vi "MOPX1 Crossover.vi"(6 "Job Selection Rule":T1, 7 "Parent 1 Schedule":u16[](array[numeric]), 8 "error in (no error)":errorcluster, 9 "Parent 2 Schedule":u16[](array[numeric]), 10 "OSSP_Problem In":refnum<class "OSSP_Problem.lvclass">, 11 "GA in":refnum<class "GA.lvclass">) -> (0 "error out":errorcluster, 1 "Child 1":T2, 2 "OSSP_Problem out":refnum<class "OSSP_Problem.lvclass">, 3 "GA out":refnum<class "GA.lvclass">, 4 "Child 2":T2)   [LabVIEW 2013, in "GA.lvclass"]
uses:
  GA.lvclass
  OSSP_Problem.lvclass
  Controls/Solution_GA.ctl
  Controls/MPOX1 Operation Selection Rule.ctl
  GA.lvclass/GA.ctl
  OSSP_Problem.lvclass/OSSP_Problem.ctl
  GanntChart_Class/Operation to Machine Job Tuple.vi
  GanntChart_Class/Check Other Machines for Schedule Time.vi
  GanntChart_Class/Schedule Job.vi
  GanntChart_Class/Find Gaps on Particular Machine.vi
  GanntChart_Class/Increment Number of Jobs on Machine.vi
  GanntChart_Class/Find Job On Other Machines.vi
  GanntChart.lvclass
panel:
  out "Child 2 Schedule":u16[](array[numeric])
  out "Child 1 Schedule":u16[](array[numeric])
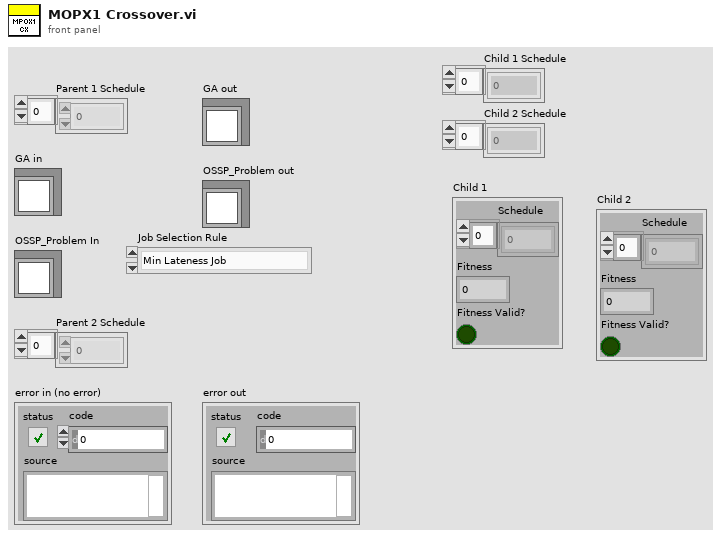
[diagram p1: front panel]
types:
  T1 = typedef "GA.lvclass/MPOX1 Operation Selection Rule.ctl" = enum16{"Min Lateness Job", "Random Job"}
  T2 = typedef "Solution_GA.ctl" = cluster{"Schedule":u16[], "Fitness":u16, "Fitness Valid?":bool}
  T3 = typedef "Scheduler Type.ctl" = enum16{"Non Delay Scheduler", "GT Active Scheduler", "FIFO Scheduler"}
  T4 = typedef "Objective.ctl" = enum16{"Makespan", "Total Tardiness"}
  T5 = typedef "GanntChart_Element.ctl" = cluster{"Operation Number":i32, "Job Number":i32, "Start Time":i32, "Procesing Time":u16, "End Time":i32}
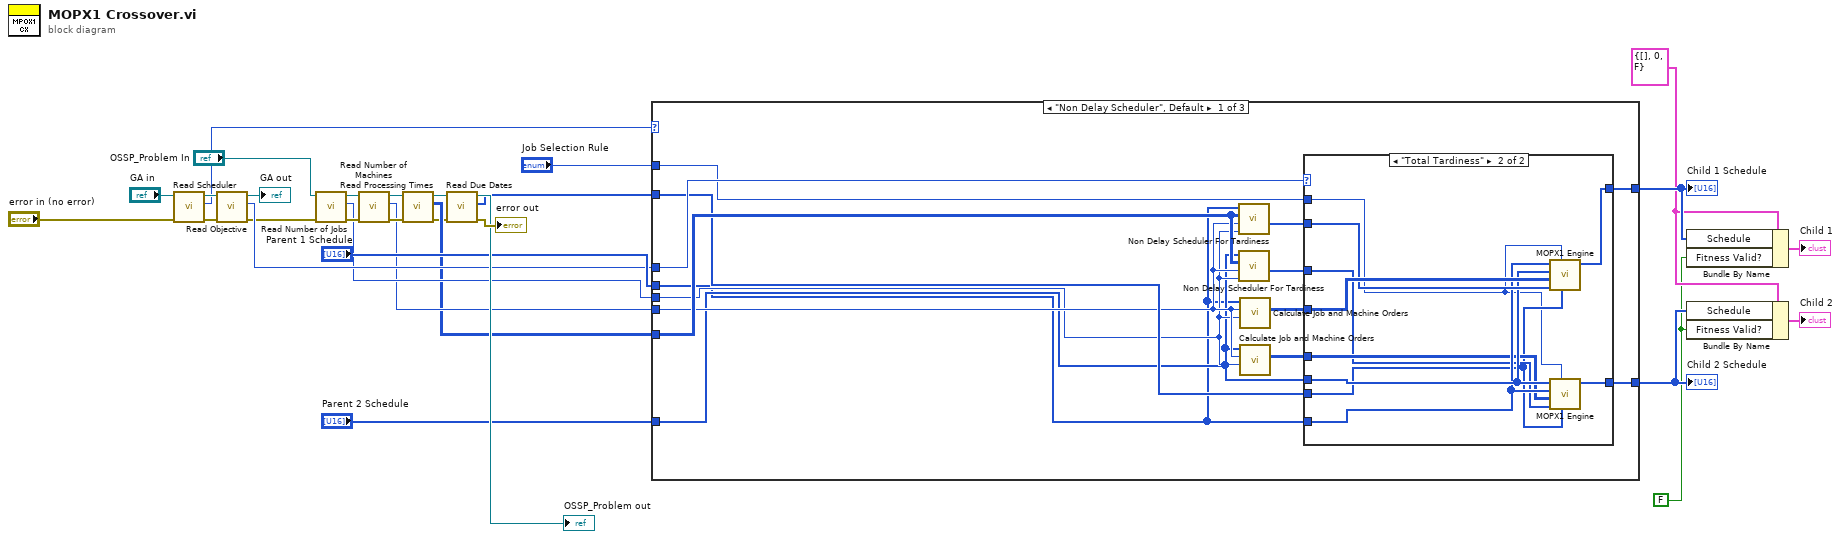
[diagram p0: block diagram]
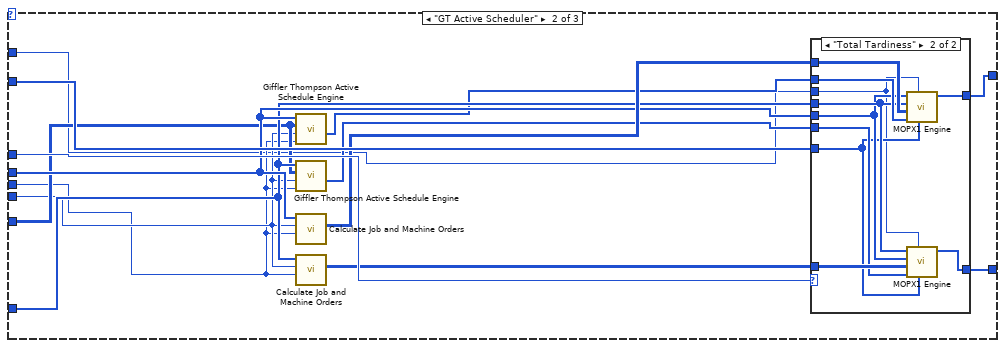
[diagram p3: hidden frame]
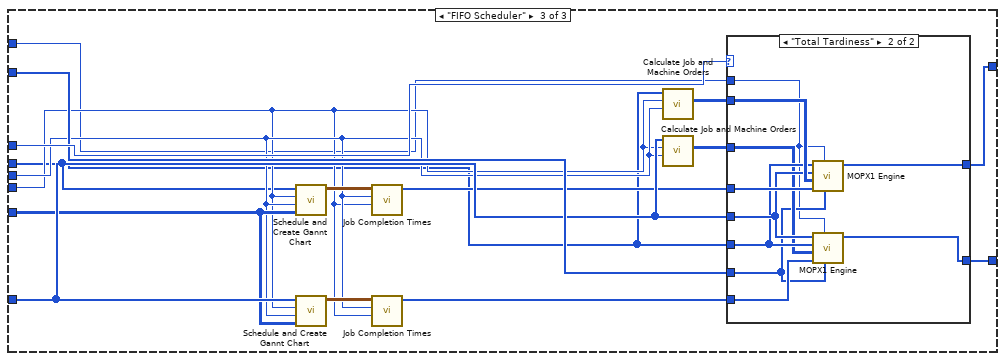
[diagram p5: hidden frame]
diagram:
  w4 = FALSE ("Fitness Valid?")
  w6 = T2 {"Schedule"=[], "Fitness"=0, "Fitness Valid?"=FALSE} ("Child 2")
  n1 = call "Read Scheduler.vi"("error in (no error)"="error in (no error)", "GA in"="GA in") -> ("error out"=w21:errorcluster, "Scheduler"=w20:T3, "GA out"=w22:refnum<class "GA.lvclass">)  [unwired: 7 in]
  n2 = call "Read Objective .vi"("error in (no error)"=w21, "GA in"=w22) -> ("error out"=w18:errorcluster, "Objective"=w19:T4, "GA out"=→"GA out":refnum<class "GA.lvclass">)  [unwired: 7 in]
  n3 = call-dynamic "Read Number of Jobs.vi"("error in (no error)"=w18, "OSSP_Problem in"="OSSP_Problem In") -> ("error out"=w17:errorcluster, "Number of Jobs"=w13:i32, "OSSP_Problem out"=w15:refnum<class "OSSP_Problem.lvclass">)  [unwired: 7 in]
  n4 = call-dynamic "Read Number of Machines.vi"("error in (no error)"=w17, "OSSP_Problem in"=w15) -> ("error out"=w16:errorcluster, "Number of Machines"=w12:i32, "OSSP_Problem out"=w14:refnum<class "OSSP_Problem.lvclass">)  [unwired: 7 in]
  n5 = call-dynamic "Read Processing Times.vi"("error in (no error)"=w16, "OSSP_Problem in"=w14) -> ("error out"=w9:errorcluster, "Processing Times"=w11:u16[][], "OSSP_Problem out"=w10:refnum<class "OSSP_Problem.lvclass">)  [unwired: 7 in]
  n6 = call "Read Due Dates.vi"("error in (no error)"=w9, "OSSP_Problem in"=w10) -> ("error out"=→"error out":errorcluster, "Due Dates"=w8:u16[], "OSSP_Problem out"=→"OSSP_Problem out":refnum<class "OSSP_Problem.lvclass">)  [unwired: 7 in]
  n7 = case shown="\"Non Delay Scheduler\", Default" w20 {
    tunnel: w19 -> [w44 w70 w98]
    tunnel: "Parent 1 Schedule" -> [w35 w67 w86]
    tunnel: "Parent 2 Schedule" -> [w36 w66 w94]
    tunnel: w13 -> [w38 w63 w91]
    tunnel: w12 -> [w39 w64 w90]
    tunnel: w11 -> [w43 w65 w92]
    tunnel: w8 -> [w42 w69 w97]
    tunnel: [w34 w59 w85] -> w7
    tunnel: [w32 w58 w84] -> w5
    tunnel: "Job Selection Rule" -> [w31 w57 w83]
    frame "Non Delay Scheduler", Default {
      n8 = call "Non Delay Scheduler For Tardiness.vi"("Number of  Jobs"=w38, "Number of Machines"=w39, "Processing Times"=w43, "Schedule"=w35) -> ("Job Completion Times"=w41:u16[])  [unwired: 3 in, 4 out]
      n9 = call "Non Delay Scheduler For Tardiness.vi"("Number of  Jobs"=w38, "Number of Machines"=w39, "Processing Times"=w43, "Schedule"=w36) -> ("Job Completion Times"=w40:u16[])  [unwired: 3 in, 4 out]
      n10 = call "Calculate Job and Machine Orders.vi"("Number of Jobs"=w38, "Number of Machines"=w39, "Schedule"=w35) -> ("MO4J"=w37:u16[][])  [unwired: 7 in, 1 out]
      n11 = call "Calculate Job and Machine Orders.vi"("Number of Jobs"=w38, "Number of Machines"=w39, "Schedule"=w36) -> ("MO4J"=w33:u16[][])  [unwired: 7 in, 1 out]
      n12 = case shown="\"Total Tardiness\"" w44 {
        tunnel: w42 -> [_ w49]
        tunnel: w41 -> [_ w54]
        tunnel: w40 -> [_ w50]
        tunnel: w37 -> [_ w55]
        tunnel: w36 -> [w45 w53]
        tunnel: w35 -> [w46 w52]
        tunnel: [w46 w56] -> w34
        tunnel: w33 -> [_ w51]
        tunnel: [w45 w48] -> w32
        tunnel: w31 -> [_ w47]
        frame "Makespan", Default {
        }
        frame "Total Tardiness" {
          n13 = call "MOPX1 Engine.vi"("Due Dates"=w49, "Job Selection Rule"=w47, "Main Parent Job Completion Times"=w54, "Main Parent  MO4J"=w55, "Secondary Parent Schedule"=w53, "Main Parent Schedule"=w52) -> ("Child Schedule"=w56:u16[])  [unwired: 5 in]
          n14 = call "MOPX1 Engine.vi"("Due Dates"=w49, "Job Selection Rule"=w47, "Main Parent Job Completion Times"=w50, "Main Parent  MO4J"=w51, "Secondary Parent Schedule"=w52, "Main Parent Schedule"=w53) -> ("Child Schedule"=w48:u16[])  [unwired: 5 in]
        }
      }
    }
    frame "GT Active Scheduler" {
      n15 = call "Giffler Thompson Active Schedule Engine.vi"("Number of  Jobs"=w63, "Number of Machines"=w64, "Processing Times"=w65, "Schedule In"=w67) -> ("Job Completion Times"=w61:u16[])  [unwired: 3 in, 4 out]
      n16 = call "Giffler Thompson Active Schedule Engine.vi"("Number of  Jobs"=w63, "Number of Machines"=w64, "Processing Times"=w65, "Schedule In"=w66) -> ("Job Completion Times"=w62:u16[])  [unwired: 3 in, 4 out]
      n17 = call "Calculate Job and Machine Orders.vi"("Number of Jobs"=w63, "Number of Machines"=w64, "Schedule"=w67) -> ("MO4J"=w68:u16[][])  [unwired: 7 in, 1 out]
      n18 = call "Calculate Job and Machine Orders.vi"("Number of Jobs"=w63, "Number of Machines"=w64, "Schedule"=w66) -> ("MO4J"=w60:u16[][])  [unwired: 7 in, 1 out]
      n19 = case shown="\"Total Tardiness\"" w70 {
        tunnel: w69 -> [_ w75]
        tunnel: w68 -> [_ w81]
        tunnel: w66 -> [w71 w79]
        tunnel: w67 -> [w72 w78]
        tunnel: [w72 w80] -> w59
        tunnel: w62 -> [_ w76]
        tunnel: w61 -> [_ w82]
        tunnel: w60 -> [_ w77]
        tunnel: [w71 w74] -> w58
        tunnel: w57 -> [_ w73]
        frame "Makespan", Default {
        }
        frame "Total Tardiness" {
          n20 = call "MOPX1 Engine.vi"("Due Dates"=w75, "Job Selection Rule"=w73, "Main Parent Job Completion Times"=w82, "Main Parent  MO4J"=w81, "Secondary Parent Schedule"=w79, "Main Parent Schedule"=w78) -> ("Child Schedule"=w80:u16[])  [unwired: 5 in]
          n21 = call "MOPX1 Engine.vi"("Due Dates"=w75, "Job Selection Rule"=w73, "Main Parent Job Completion Times"=w76, "Main Parent  MO4J"=w77, "Secondary Parent Schedule"=w78, "Main Parent Schedule"=w79) -> ("Child Schedule"=w74:u16[])  [unwired: 5 in]
        }
      }
    }
    frame "FIFO Scheduler" {
      n22 = call "Schedule and Create Gannt Chart.vi"("Processing Times (Rows Mach.Cols Jobs)"=w92, "Number of Jobs"=w91, "Number of Machines"=w90, "Schedule"=w86) -> ("Gannt Chart Out"=w95:T5[][])  [unwired: 6 in, 1 out]
      n23 = call "Schedule and Create Gannt Chart.vi"("Processing Times (Rows Mach.Cols Jobs)"=w92, "Number of Jobs"=w91, "Number of Machines"=w90, "Schedule"=w94) -> ("Gannt Chart Out"=w93:T5[][])  [unwired: 6 in, 1 out]
      n24 = call "Job Completion Times.vi"("Number Of Machines"=w90, "Number Of Jobs"=w91, "Gannt Chart In"=w95) -> ("Job Completion Times"=w89:u16[])  [unwired: 8 in]
      n25 = call "Job Completion Times.vi"("Number Of Machines"=w90, "Number Of Jobs"=w91, "Gannt Chart In"=w93) -> ("Job Completion Times"=w88:u16[])  [unwired: 8 in]
      n26 = call "Calculate Job and Machine Orders.vi"("Number of Jobs"=w91, "Number of Machines"=w90, "Schedule"=w86) -> ("MO4J"=w96:u16[][])  [unwired: 7 in, 1 out]
      n27 = call "Calculate Job and Machine Orders.vi"("Number of Jobs"=w91, "Number of Machines"=w90, "Schedule"=w94) -> ("MO4J"=w87:u16[][])  [unwired: 7 in, 1 out]
      n28 = case shown="\"Total Tardiness\"" w98 {
        tunnel: w97 -> [_ w103]
        tunnel: w96 -> [_ w109]
        tunnel: w94 -> [w99 w107]
        tunnel: w86 -> [w100 w106]
        tunnel: [w100 w108] -> w85
        tunnel: w89 -> [_ w110]
        tunnel: w88 -> [_ w104]
        tunnel: w87 -> [_ w105]
        tunnel: [w99 w102] -> w84
        tunnel: w83 -> [_ w101]
        frame "Makespan", Default {
        }
        frame "Total Tardiness" {
          n29 = call "MOPX1 Engine.vi"("Due Dates"=w103, "Job Selection Rule"=w101, "Main Parent Job Completion Times"=w110, "Main Parent  MO4J"=w109, "Secondary Parent Schedule"=w107, "Main Parent Schedule"=w106) -> ("Child Schedule"=w108:u16[])  [unwired: 5 in]
          n30 = call "MOPX1 Engine.vi"("Due Dates"=w103, "Job Selection Rule"=w101, "Main Parent Job Completion Times"=w104, "Main Parent  MO4J"=w105, "Secondary Parent Schedule"=w106, "Main Parent Schedule"=w107) -> ("Child Schedule"=w102:u16[])  [unwired: 5 in]
        }
      }
    }
  }
  "Child 1 Schedule" <- w7
  "Child 2 Schedule" <- w5
  n31 = Bundle By Name(cluster=w6, "Schedule"=w7, "Fitness Valid?"=w4) -> (→"Child 1":T2)
  n32 = Bundle By Name(cluster=w6, "Schedule"=w5, "Fitness Valid?"=w4) -> (→"Child 2":T2)
